vi "Create Message Queue.vi"(6 "Flush (F)":bool, 7 "max queue size (-1, unlimited)":i32=-1, 8 "error in (no error)":errorcluster, 11 "Queue Name":string) -> (0 "error out":errorcluster, 2 "created new?":bool, 3 "queue ref out":T1)   [LabVIEW 2013, in "Interloop MessageQ.lvlib"]
doc: "Creates a new message queue and adds it to the message queue manager."
uses:
  Interloop MessageQ.lvlib
  Message Queue Ref.ctl
  Message cluster.ctl
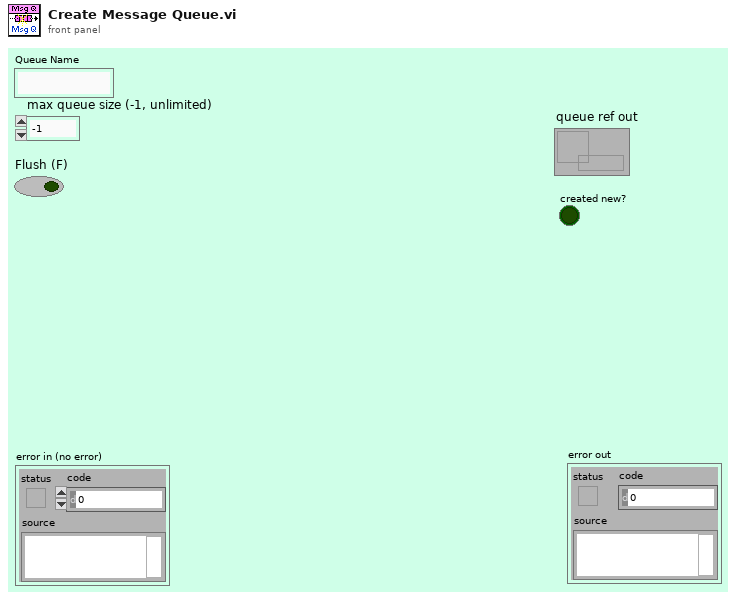
[diagram p1: front panel]
types:
  T1 = typedef "Interloop MessageQ.lvlib/Message Queue Ref.ctl" = refnum<queue>
  T2 = typedef "Interloop MessageQ.lvlib/Message cluster.ctl" = cluster{"Message String":string, "Data":variant}
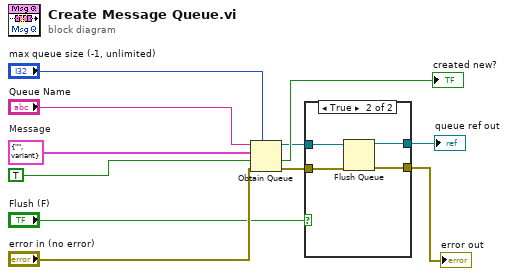
[diagram p0: block diagram]
diagram:
  w5 = T2 {"Message String"="", "Data"=variant}  # Message
  n1 = Obtain Queue(max queue size (-1, unlimited)="max queue size (-1, unlimited)", name (unnamed)="Queue Name", element data type=w5, create if not found? (T)=TRUE, error in (no error)="error in (no error)") -> (queue out=w6:refnum<queue>, created new?=→"created new?":bool, error out=w8:errorcluster)
  n2 = case shown="True" "Flush (F)" {
    tunnel: w8 -> [w12 w17]
    tunnel: [w12 w16] -> w7
    tunnel: w6 -> [w13 w15]
    tunnel: [w13 w14] -> w1
    frame False {
    }
    frame True {
      n3 = Flush Queue(queue=w15, error in (no error)=w17) -> (queue out=w14:refnum<queue>, error out=w16:errorcluster)  [unwired: 1 out]
    }
  }
  "error out" <- w7
  "queue ref out" <- w1
